vi "GDSString_RemoveBaseMethodCallString.vi"(11 "Method Call String":string) -> (3 "Base call Removed":string)   [LabVIEW 2016]
uses:
  <vilib>/Utility/error.llb/whitespace.ctl
panel:
  out "Base call arguments text":string
  out "BaseClassCallRemoved":bool
  # "public AddCommand(IReciever reciever)\n        : base (reciever)"
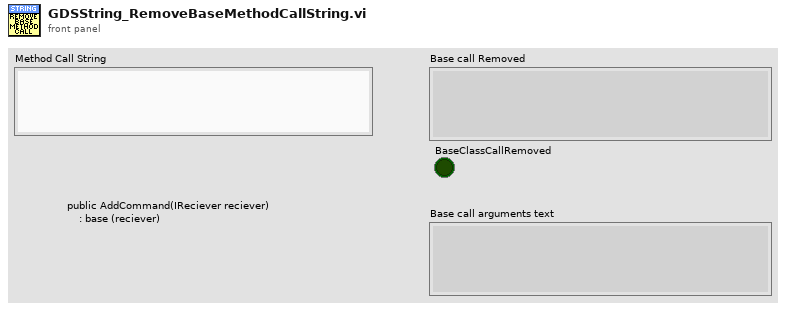
[diagram p1: front panel]
types:
  T1 = typedef "whitespace.ctl" = u16
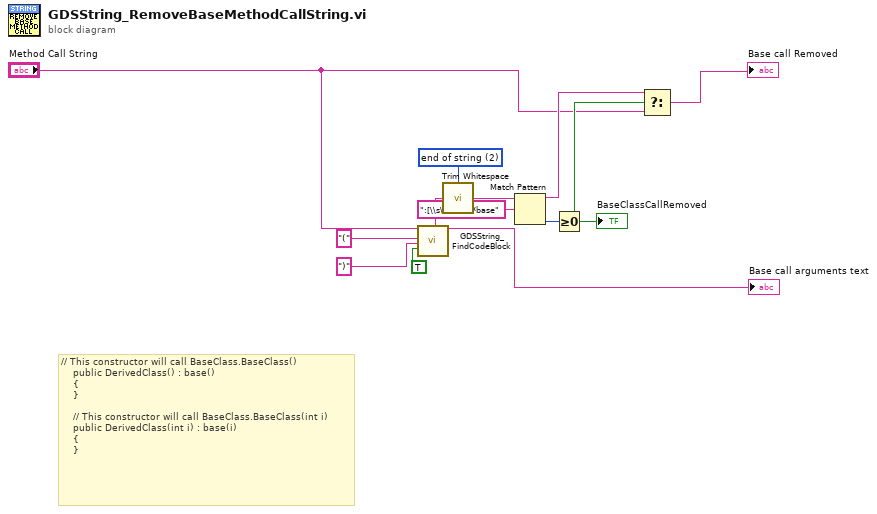
[diagram p0: block diagram]
diagram:
  w7 = T1 2 items=["both", "start of string", "end of string"] ("location (both)")
  # "// This constructor will call BaseClass.BaseClass() \n    public DerivedClass() : base()\n    {\n    }\n\n    // This constructor will call BaseClass.BaseClass(int i) \n    public DerivedClass(int i) : base(i)\n    {\n    }"
  n1 = call <resource>:"GDSString_FindCodeBlock.vi"("Text"="Method Call String", "CodeBlockStartCharacter( { )"="(", "CodeBlockEndCharacter( } )"=")", "Search Backwards"=TRUE) -> ("TextBeforeBlock"=w10:string, "BlockText"=→"Base call arguments text":string)  [unwired: 7 in, 7 out]
  n2 = call <vilib>:"Trim Whitespace.vi"("string"=w10, "location (both)"=w7) -> ("trimmed string"=w8:string)
  n3 = Match Pattern(string=w8, regular expression=":[\\s\\n\\r\\t]*base") -> (before substring=w4:string, offset past match=w6:i32)  [unwired: 1 in, 2 out]
  n4 = Greater Or Equal To 0?(x=w6) -> (x >= 0?=w5:bool)
  "BaseClassCallRemoved" <- w5
  n5 = Select(t=w4, s=w5, f="Method Call String") -> (s? t:f=→"Base call Removed":string)
